vi "WhitePlot.vi"(11 "Paths":path[](array[path])=[path "/Users/crogers/Desktop/Ted/Ob16 Galahue Plowden 2013 H_Ave.trf"]) -> ()   [LabVIEW 2022 SP3]
uses:
  Perspective/subs/Perspective_Globals.vi
panel:
  in  "signal type":T1(ring)=enum."Sawtooth Wave"
  in  "# harmonics":i32=40
  in  "# freq":i32=48
  out "Graph":picture
  in  "Files":u16(ring) items=["1741 del G. HV 20 V_007.trf", "1741 del G. HV 20 V_007.trf", "1741 del G. HV 20 V_008.trf", "1741 del G. HV 20 V_008.trf", "1741 del G. HV 20 V_009.trf", "1741 del G. HV 20 V_009.trf", "1741 del G. HV 20 V_010.trf", "1741 del G. HV 20 V_010.trf", "1741 del G. HV 20 V_011.trf"]
  out "Slice":dbl[](graph)=[29.445158043811198, 36.55833093424573, 40.44091855599027, 37.67653983236719, 3.901363084528417, 43.245886090198724, 36.36206724043218, 58.6607561868737, 51.19267039727471, 16.66678219935681, 46.372145605984485, 40.65058675099788, -0.1217403502671347, 38.33577783712102, 35.852538445709634, 29.35326642077404, 49.768103526439276, 44.09040502089316, 26.44794576028672, 43.78480234185166, 12.786831883362723, nan, nan, nan, nan, nan, nan, nan, nan, nan, nan, nan, nan, nan, nan, nan, nan, nan, nan, nan]
  in  "Smoothing":u16(ring) items=["No smoothing"=0, "1/4 semitone"=25, "1/2 semitone"=50, "1 semitone"=100, "2 semitones"=200, "3 semitones"=300, "4 semitones"=400, "Octave"=1200]
  in  "Color Table":T2(ring)=enum."Rainbow"
  out "TRF":cluster{dbl, "df":dbl, dbl[]}(graph)={199.951171875, "df"=0.732421875, array[13381 elements]}
  out "2D Plot":dbl[][](graph)=[[nan, 20.049987226429913, 25.054902961250857, 29.445158043811198, 34.46385501795731, 44.780627225419565, 51.406191185965646, 49.67631609372249, 40.709611963732584, 38.92269108407762, 40.35029451326228, 33.055745098571954, 41.52467260523725, 39.21617102292643, 15.173302135246772, 40.695109109084115, 42.444899082336, 56.77593405896198, 51.382201329207334, 43.21477455890306, 50.80370011373546, 35.98612449368547, 47.77204513443894, 30.857881410259274, 46.643671439889445, 47.49403661581599, -1.4346363375750995, 19.0211768965106, 45.28695989710588, 40.69907700152897, 46.376353342172045, 39.045432783467874, 48.20425730785347, 35.99159002094946, 35.20324613314526, 51.91563451765467, 18.854037759092634, 37.28439063047342, -19.57168106597702, 25.22610299025189, 29.263013635587455, 30.82063676591259, 33.55395737125039, 18.19981181386353, 24.102157288646847, 39.34971755858826, 22.241809662116708, 68.52224965159985], [54.26627490024298, 47.12526752661166, 56.85500723817575, 36.55833093424573, 38.634265924869595, 51.93988341853376, 45.638032395871505, 66.45923338856223, 48.341086236955675, 44.73549896684294, 82.8746731094306, 36.13504669577988, 32.4985458705831, 38.46882120330299, 25.627379738354886, 38.640118352136994, 69.51016913200667, 47.08441844740895, 43.538098543664844, 37.74770538349388, 2.607749244145145, 35.43065545900197, 48.78584596653637, 44.50117153673708, 47.18149466094815, 37.167565780443084, -11.290057999008061, 38.82305284871714, 34.622338104545236, 45.77689163136356, 27.988762535569126, 35.05040002787151, 46.39143083402964, 41.744798474139316, 32.89651926775419, 62.34466322011301, 39.44356696797309, 46.6442728756223, -10.828073640077598, 26.81232522566393, 48.71727144928745, 32.03610040569839, 72.79095309960253, 36.67913423432094, 48.058266713190754, nan, nan, nan], [53.04185758812355, 84.71388448770111, 17.51080377410179, 40.44091855599027, 39.91331658353087, 28.362665427675545, 55.229556863313356, 56.42371074485528, 47.76931799964777, 39.97049168305633, 57.15726261780386, 37.542352295940155, 44.21162796738528, 17.48325982608004, 40.43782874904303, 38.742739205630784, 46.032627402046785, 20.05630274646011, 45.78665416858822, 35.24520049827762, 39.158716639789034, 11.924005690223789, 29.897529283546916, 33.60264045829483, 31.392790303731708, 19.506700819440113, -9.215795080095525, 50.42813350565264, 32.59479614372741, 31.01757424069985, 42.71237559822864, 51.983617982184924, 34.35731157695301, 42.627623260331376, 19.10147623463881, 54.50616438544329, 18.296402637224976, 58.61753732987064, nan, nan, nan, nan, nan, nan, nan, nan, nan, nan], [39.51596652723599, 29.184271442763787, 16.957827346664814, 37.67653983236719, 63.59782300125275, 48.322834414258296, 40.39060448678149, 38.07851466585304, 52.219678596166396, 61.51482106592874, 46.8634576004301, 37.06553982367735, 38.09179565041872, 11.208063972191031, 54.731123202538576, 29.039234290370757, 34.051601948841004, 41.1260225901982, 52.08899147984912, 28.05180790327435, 34.07973803463468, 42.3996411700281, 20.192703080247497, 56.168607595418976, 33.25620455392025, 39.61259618090587, 1.6416847986202243, 24.841476380656804, 37.55245428572219, 27.459839855335257, 66.77063240632266, 36.5729389128255, 41.814287416945945, nan, nan, nan, nan, nan, nan, nan, nan, nan, nan, nan, nan, nan, nan, nan], [48.16850062624863, 42.24542108686359, 44.340073178907026, 3.901363084528417, 42.347676492963295, 41.98102702804944, 32.095730941153256, 7.619084984059836, 32.35066397625168, 32.29142786493228, 40.21124807070387, 14.63732432854075, 64.87319042636963, 3.8937001997797758, 42.35230450100133, 14.130476829463692, 28.642057668910525, 38.68345012614008, 40.520552066845205, 52.826865227382584, 27.4036034714791, 73.37393650330726, 10.947826509906172, 39.440434175724384, 31.785624530969287, 39.726239419396016, 27.00365963632292, 17.381561857680012, 36.93147689751727, nan, nan, nan, nan, nan, nan, nan, nan, nan, nan, nan, nan, nan, nan, nan, nan, nan, nan, nan], [35.60423156346238, 46.08009523979531, 36.87411957248013, 43.245886090198724, 41.3473179130062, 26.344792341973875, 41.08933756077456, 27.303763144444684, 32.28100773510765, 34.38861713258833, 31.00322874795537, 55.966772111396814, 33.80384369988236, 22.921989435884473, 8.945740357752978, 42.39269732229077, 33.87217699897191, 33.14532562541018, 33.524294370197566, 44.041506495823185, 37.757502066680686, 41.939614181516674, 8.546073278104322, 48.000016608061514, 35.00765134648421, 51.85386377302325, nan, nan, nan, nan, nan, nan, nan, nan, nan, nan, nan, nan, nan, nan, nan, nan, nan, nan, nan, nan, nan, nan], [32.61310636745673, 38.97527846530624, 35.641622198785086, 36.36206724043218, 27.795949148894337, 54.187637574190326, 36.401734072540044, 30.917571343879366, 37.20179247250486, 27.793291744454113, 25.775060428523826, 10.666225801452157, 38.49962709844564, 11.781027471364073, 13.761017548356374, 42.53126220573978, 35.128829087408405, 40.161072813389424, 41.09343386515138, 35.9780075897034, 17.001024691654287, 42.92404272966259, 26.64675831650957, nan, nan, nan, nan, nan, nan, nan, nan, nan, nan, nan, nan, nan, nan, nan, nan, nan, nan, nan, nan, nan, nan, nan, nan, nan], [29.681571025848356, 42.60929144128346, 48.67052729500847, 58.6607561868737, 33.95354038216709, 41.11614535668331, 47.65431912163869, -11.009770350280277, 36.94947500875874, 39.83841719056124, 31.381560080516877, 52.500057048302736, 38.174458325750436, 20.80842003831775, 12.283677007960899, 35.16227099829001, 59.770944975043896, 21.937359659167246, 60.53209358540707, 36.682904986845664, 39.7581113435772, nan, nan, nan, nan, nan, nan, nan, nan, nan, nan, nan, nan, nan, nan, nan, nan, nan, nan, nan, nan, nan, nan, nan, nan, nan, nan, nan], [40.464054607466934, 37.58597485171173, 39.87038706581357, 51.19267039727471, 37.67639985297179, 23.13937723997912, 37.55595835553924, 42.4209222579333, 42.27910760517511, 30.522265980669758, 26.136408931304445, -2.9872106006803496, 31.322538117444275, 2.9044348449634656, 3.5797530867064515, 50.092277015634636, 38.50977087060315, 47.533818499292835, 35.62939006713031, nan, nan, nan, nan, nan, nan, nan, nan, nan, nan, nan, nan, nan, nan, nan, nan, nan, nan, nan, nan, nan, nan, nan, nan, nan, nan, nan, nan, nan], [58.5659239452997, 26.982848813621306, 36.31906856692317, 16.66678219935681, 49.49109923197512, 40.11411668922503, 37.75341628139453, 48.30992190831356, 49.081010121114915, 61.181425385472934, 22.430170217674966, 48.6155340973561, 32.675460627661636, 13.916675441379617, 21.021585447450946, 49.25166283256742, 62.27105544588605, nan, nan, nan, nan, nan, nan, nan, nan, nan, nan, nan, nan, nan, nan, nan, nan, nan, nan, nan, nan, nan, nan, nan, nan, nan, nan, nan, nan, nan, nan, nan], [54.412382522142494, 36.137207842053776, 2.764148858981666, 46.372145605984485, 37.243085887419376, 34.537737023825855, 55.257207308976035, 51.464533050016435, 39.80085824725523, 44.11810710124637, 34.10663843132296, 5.979096794947166, 25.782557120064702, 30.561510305365577, 40.94721364933057, nan, nan, nan, nan, nan, nan, nan, nan, nan, nan, nan, nan, nan, nan, nan, nan, nan, nan, nan, nan, nan, nan, nan, nan, nan, nan, nan, nan, nan, nan, nan, nan, nan], [31.369910198236113, 37.07152928092298, 10.648427094010238, 40.65058675099788, 23.51231403437172, 27.206691169768323, 36.277462506216686, 34.08022467450811, 35.763375497264654, 29.232268970303785, 23.380681094116376, 44.186129447967446, 35.05238954844841, 50.27126063942963, nan, nan, nan, nan, nan, nan, nan, nan, nan, nan, nan, nan, nan, nan, nan, nan, nan, nan, nan, nan, nan, nan, nan, nan, nan, nan, nan, nan, nan, nan, nan, nan, nan, nan], [47.82026138668182, 33.43812207351204, 25.299758140785883, -0.1217403502671347, 22.16453525325594, 48.48725544404082, 42.08447575914906, 19.62567783478579, 38.80170108501365, 40.192102073325636, 33.03273363219364, 36.03429599678489, 28.409628306750335, nan, nan, nan, nan, nan, nan, nan, nan, nan, nan, nan, nan, nan, nan, nan, nan, nan, nan, nan, nan, nan, nan, nan, nan, nan, nan, nan, nan, nan, nan, nan, nan, nan, nan, nan], [38.74276193034642, 51.348432885653914, 32.25091267120466, 38.33577783712102, 29.752691953524675, 38.079351040376174, 38.87949376223, 0.26530157389657355, 29.509618670886084, 40.33082643082275, 34.24093489901787, nan, nan, nan, nan, nan, nan, nan, nan, nan, nan, nan, nan, nan, nan, nan, nan, nan, nan, nan, nan, nan, nan, nan, nan, nan, nan, nan, nan, nan, nan, nan, nan, nan, nan, nan, nan, nan], [38.005167377161804, 31.69088276912158, 52.845640027356204, 35.852538445709634, 43.1225994596063, 37.243651148967345, 29.029508255433182, 9.006139857266586, 38.32944523498376, 36.834360308878054, nan, nan, nan, nan, nan, nan, nan, nan, nan, nan, nan, nan, nan, nan, nan, nan, nan, nan, nan, nan, nan, nan, nan, nan, nan, nan, nan, nan, nan, nan, nan, nan, nan, nan, nan, nan, nan, nan], [35.90269660816785, 39.364578709379494, 39.55419749173399, 29.35326642077404, 53.69867614237862, 31.967502560639367, 54.7193336975603, 30.88778141801589, 39.34981484445568, nan, nan, nan, nan, nan, nan, nan, nan, nan, nan, nan, nan, nan, nan, nan, nan, nan, nan, nan, nan, nan, nan, nan, nan, nan, nan, nan, nan, nan, nan, nan, nan, nan, nan, nan, nan, nan, nan, nan], [36.30638411087302, 25.09057920682725, 45.46164717529554, 49.768103526439276, 23.289405968677816, 49.15198590837125, 35.1560324577208, 42.864683043159424, nan, nan, nan, nan, nan, nan, nan, nan, nan, nan, nan, nan, nan, nan, nan, nan, nan, nan, nan, nan, nan, nan, nan, nan, nan, nan, nan, nan, nan, nan, nan, nan, nan, nan, nan, nan, nan, nan, nan, nan], [31.462436582201292, 30.362788351721534, 36.81834627839507, 44.09040502089316, 33.57068005060175, 32.74557557265104, 39.515790233414656, nan, nan, nan, nan, nan, nan, nan, nan, nan, nan, nan, nan, nan, nan, nan, nan, nan, nan, nan, nan, nan, nan, nan, nan, nan, nan, nan, nan, nan, nan, nan, nan, nan, nan, nan, nan, nan, nan, nan, nan, nan], [34.58411077100862, 33.23559013285732, -5.662822029697699, 26.44794576028672, 35.487431815874324, 40.942138140629154, nan, nan, nan, nan, nan, nan, nan, nan, nan, nan, nan, nan, nan, nan, nan, nan, nan, nan, nan, nan, nan, nan, nan, nan, nan, nan, nan, nan, nan, nan, nan, nan, nan, nan, nan, nan, nan, nan, nan, nan, nan, nan], [34.61465926871371, 17.18392844569568, 13.031570274998831, 43.78480234185166, 56.1573881112846, nan, nan, nan, nan, nan, nan, nan, nan, nan, nan, nan, nan, nan, nan, nan, nan, nan, nan, nan, nan, nan, nan, nan, nan, nan, nan, nan, nan, nan, nan, nan, nan, nan, nan, nan, nan, nan, nan, nan, nan, nan, nan, nan], [29.186029345513607, 47.978737915500574, 17.360000383750858, 12.786831883362723, nan, nan, nan, nan, nan, nan, nan, nan, nan, nan, nan, nan, nan, nan, nan, nan, nan, nan, nan, nan, nan, nan, nan, nan, nan, nan, nan, nan, nan, nan, nan, nan, nan, nan, nan, nan, nan, nan, nan, nan, nan, nan, nan, nan], [25.72159338389789, 36.84666611970028, 34.76691669928632, nan, nan, nan, nan, nan, nan, nan, nan, nan, nan, nan, nan, nan, nan, nan, nan, nan, nan, nan, nan, nan, nan, nan, nan, nan, nan, nan, nan, nan, nan, nan, nan, nan, nan, nan, nan, nan, nan, nan, nan, nan, nan, nan, nan, nan], [27.424976418713154, 38.48369817799687, 50.658137928834435, nan, nan, nan, nan, nan, nan, nan, nan, nan, nan, nan, nan, nan, nan, nan, nan, nan, nan, nan, nan, nan, nan, nan, nan, nan, nan, nan, nan, nan, nan, nan, nan, nan, nan, nan, nan, nan, nan, nan, nan, nan, nan, nan, nan, nan], [34.75082504002703, 44.286747839093266, nan, nan, nan, nan, nan, nan, nan, nan, nan, nan, nan, nan, nan, nan, nan, nan, nan, nan, nan, nan, nan, nan, nan, nan, nan, nan, nan, nan, nan, nan, nan, nan, nan, nan, nan, nan, nan, nan, nan, nan, nan, nan, nan, nan, nan, nan], [35.40073024186071, nan, nan, nan, nan, nan, nan, nan, nan, nan, nan, nan, nan, nan, nan, nan, nan, nan, nan, nan, nan, nan, nan, nan, nan, nan, nan, nan, nan, nan, nan, nan, nan, nan, nan, nan, nan, nan, nan, nan, nan, nan, nan, nan, nan, nan, nan, nan], [28.955349958389448, nan, nan, nan, nan, nan, nan, nan, nan, nan, nan, nan, nan, nan, nan, nan, nan, nan, nan, nan, nan, nan, nan, nan, nan, nan, nan, nan, nan, nan, nan, nan, nan, nan, nan, nan, nan, nan, nan, nan, nan, nan, nan, nan, nan, nan, nan, nan], [nan, nan, nan, nan, nan, nan, nan, nan, nan, nan, nan, nan, nan, nan, nan, nan, nan, nan, nan, nan, nan, nan, nan, nan, nan, nan, nan, nan, nan, nan, nan, nan, nan, nan, nan, nan, nan, nan, nan, nan, nan, nan, nan, nan, nan, nan, nan, nan], [nan, nan, nan, nan, nan, nan, nan, nan, nan, nan, nan, nan, nan, nan, nan, nan, nan, nan, nan, nan, nan, nan, nan, nan, nan, nan, nan, nan, nan, nan, nan, nan, nan, nan, nan, nan, nan, nan, nan, nan, nan, nan, nan, nan, nan, nan, nan, nan], [nan, nan, nan, nan, nan, nan, nan, nan, nan, nan, nan, nan, nan, nan, nan, nan, nan, nan, nan, nan, nan, nan, nan, nan, nan, nan, nan, nan, nan, nan, nan, nan, nan, nan, nan, nan, nan, nan, nan, nan, nan, nan, nan, nan, nan, nan, nan, nan], [nan, nan, nan, nan, nan, nan, nan, nan, nan, nan, nan, nan, nan, nan, nan, nan, nan, nan, nan, nan, nan, nan, nan, nan, nan, nan, nan, nan, nan, nan, nan, nan, nan, nan, nan, nan, nan, nan, nan, nan, nan, nan, nan, nan, nan, nan, nan, nan], [nan, nan, nan, nan, nan, nan, nan, nan, nan, nan, nan, nan, nan, nan, nan, nan, nan, nan, nan, nan, nan, nan, nan, nan, nan, nan, nan, nan, nan, nan, nan, nan, nan, nan, nan, nan, nan, nan, nan, nan, nan, nan, nan, nan, nan, nan, nan, nan], [nan, nan, nan, nan, nan, nan, nan, nan, nan, nan, nan, nan, nan, nan, nan, nan, nan, nan, nan, nan, nan, nan, nan, nan, nan, nan, nan, nan, nan, nan, nan, nan, nan, nan, nan, nan, nan, nan, nan, nan, nan, nan, nan, nan, nan, nan, nan, nan], [nan, nan, nan, nan, nan, nan, nan, nan, nan, nan, nan, nan, nan, nan, nan, nan, nan, nan, nan, nan, nan, nan, nan, nan, nan, nan, nan, nan, nan, nan, nan, nan, nan, nan, nan, nan, nan, nan, nan, nan, nan, nan, nan, nan, nan, nan, nan, nan], [nan, nan, nan, nan, nan, nan, nan, nan, nan, nan, nan, nan, nan, nan, nan, nan, nan, nan, nan, nan, nan, nan, nan, nan, nan, nan, nan, nan, nan, nan, nan, nan, nan, nan, nan, nan, nan, nan, nan, nan, nan, nan, nan, nan, nan, nan, nan, nan], [nan, nan, nan, nan, nan, nan, nan, nan, nan, nan, nan, nan, nan, nan, nan, nan, nan, nan, nan, nan, nan, nan, nan, nan, nan, nan, nan, nan, nan, nan, nan, nan, nan, nan, nan, nan, nan, nan, nan, nan, nan, nan, nan, nan, nan, nan, nan, nan], [nan, nan, nan, nan, nan, nan, nan, nan, nan, nan, nan, nan, nan, nan, nan, nan, nan, nan, nan, nan, nan, nan, nan, nan, nan, nan, nan, nan, nan, nan, nan, nan, nan, nan, nan, nan, nan, nan, nan, nan, nan, nan, nan, nan, nan, nan, nan, nan], [nan, nan, nan, nan, nan, nan, nan, nan, nan, nan, nan, nan, nan, nan, nan, nan, nan, nan, nan, nan, nan, nan, nan, nan, nan, nan, nan, nan, nan, nan, nan, nan, nan, nan, nan, nan, nan, nan, nan, nan, nan, nan, nan, nan, nan, nan, nan, nan], [nan, nan, nan, nan, nan, nan, nan, nan, nan, nan, nan, nan, nan, nan, nan, nan, nan, nan, nan, nan, nan, nan, nan, nan, nan, nan, nan, nan, nan, nan, nan, nan, nan, nan, nan, nan, nan, nan, nan, nan, nan, nan, nan, nan, nan, nan, nan, nan], [nan, nan, nan, nan, nan, nan, nan, nan, nan, nan, nan, nan, nan, nan, nan, nan, nan, nan, nan, nan, nan, nan, nan, nan, nan, nan, nan, nan, nan, nan, nan, nan, nan, nan, nan, nan, nan, nan, nan, nan, nan, nan, nan, nan, nan, nan, nan, nan], [nan, nan, nan, nan, nan, nan, nan, nan, nan, nan, nan, nan, nan, nan, nan, nan, nan, nan, nan, nan, nan, nan, nan, nan, nan, nan, nan, nan, nan, nan, nan, nan, nan, nan, nan, nan, nan, nan, nan, nan, nan, nan, nan, nan, nan, nan, nan, nan]]
  out "size(s)":i32=65
  # "Plotting Energy At Overtones"
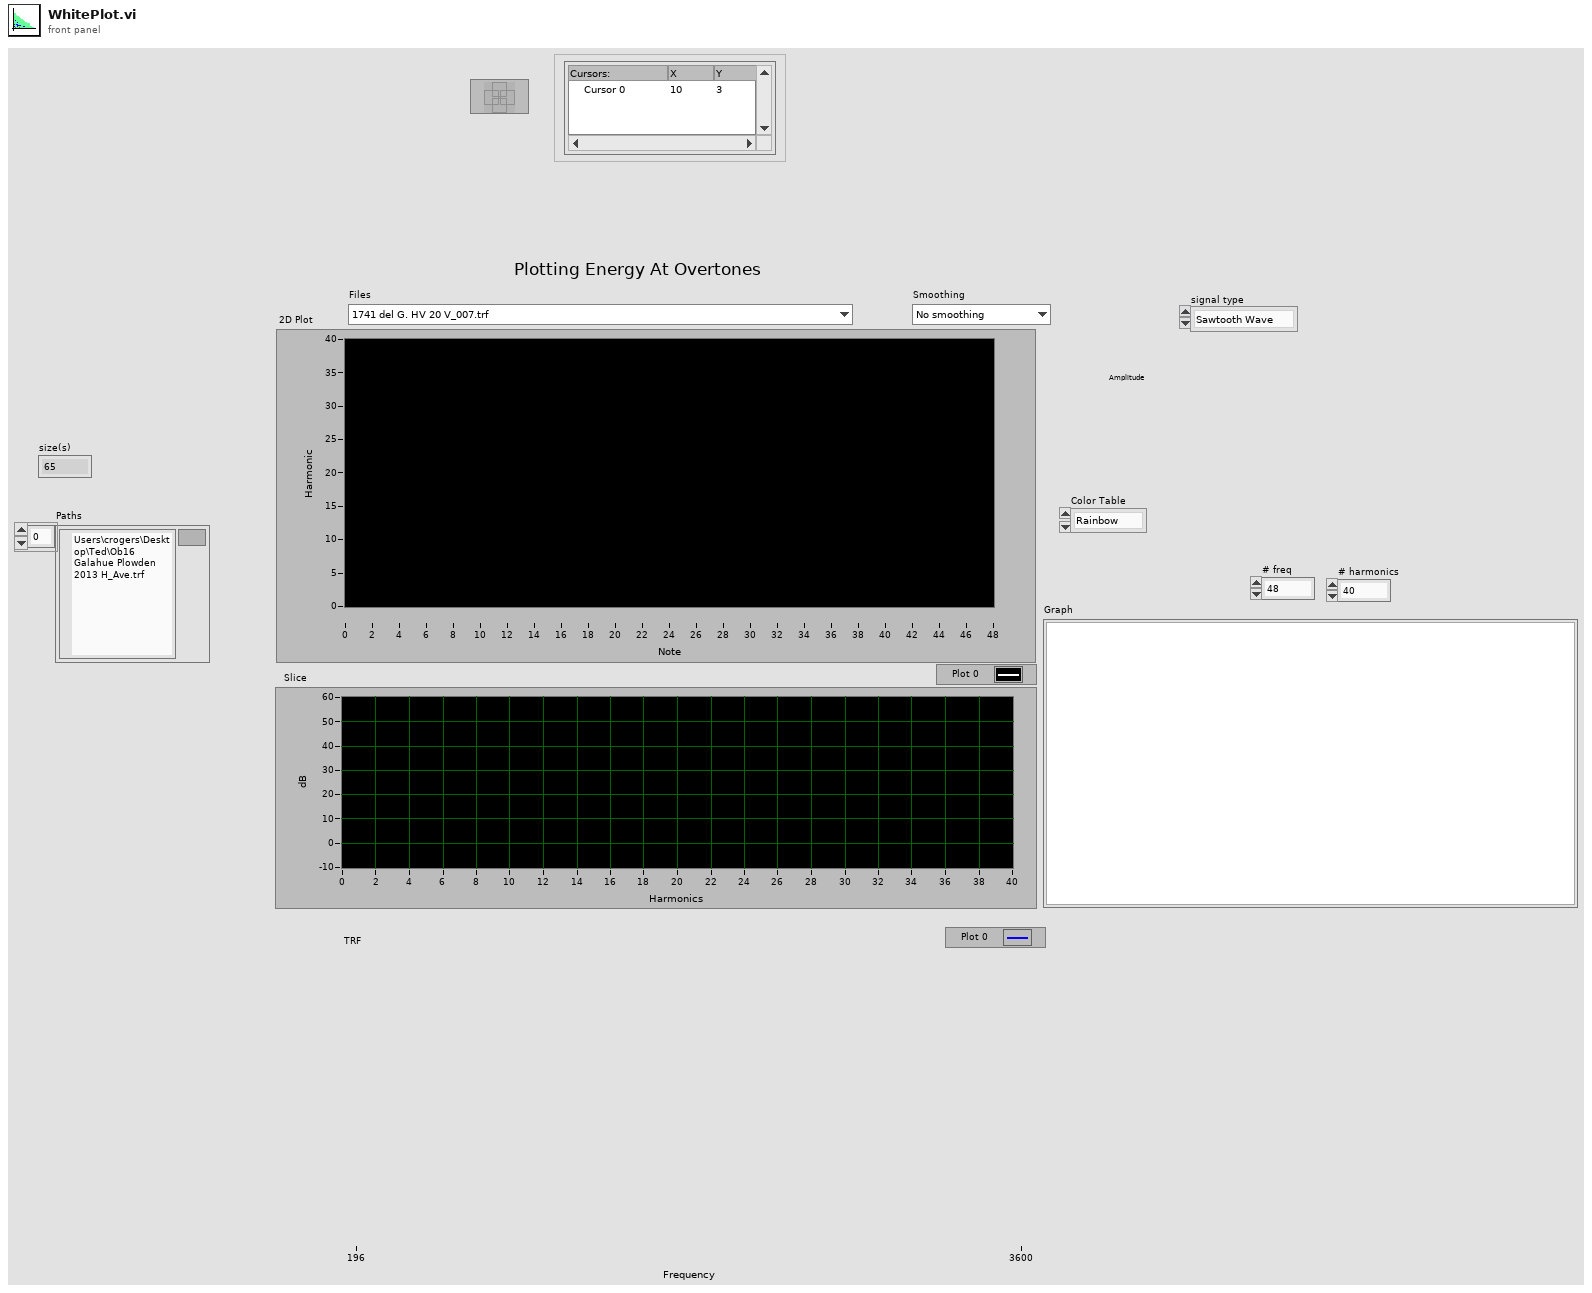
[diagram p1: front panel]
types:
  T1 = enum16{"Sine Wave", "Triangle Wave", "Square Wave", "Sawtooth Wave"}
  T2 = enum16{"Apricot", "Carnation", "Ether", "Greyscale", "Greyscale-banded", "Hot Metal", "Lava Waves", "Mac", "Morning Glory", "Rainbow", "Rainbow-banded", "Rainbow-inverted", "Rainbow-striped", "Saturn", "Seismic", "Space"}
  T3 = cluster{"Notes":string, "format string":string}[]
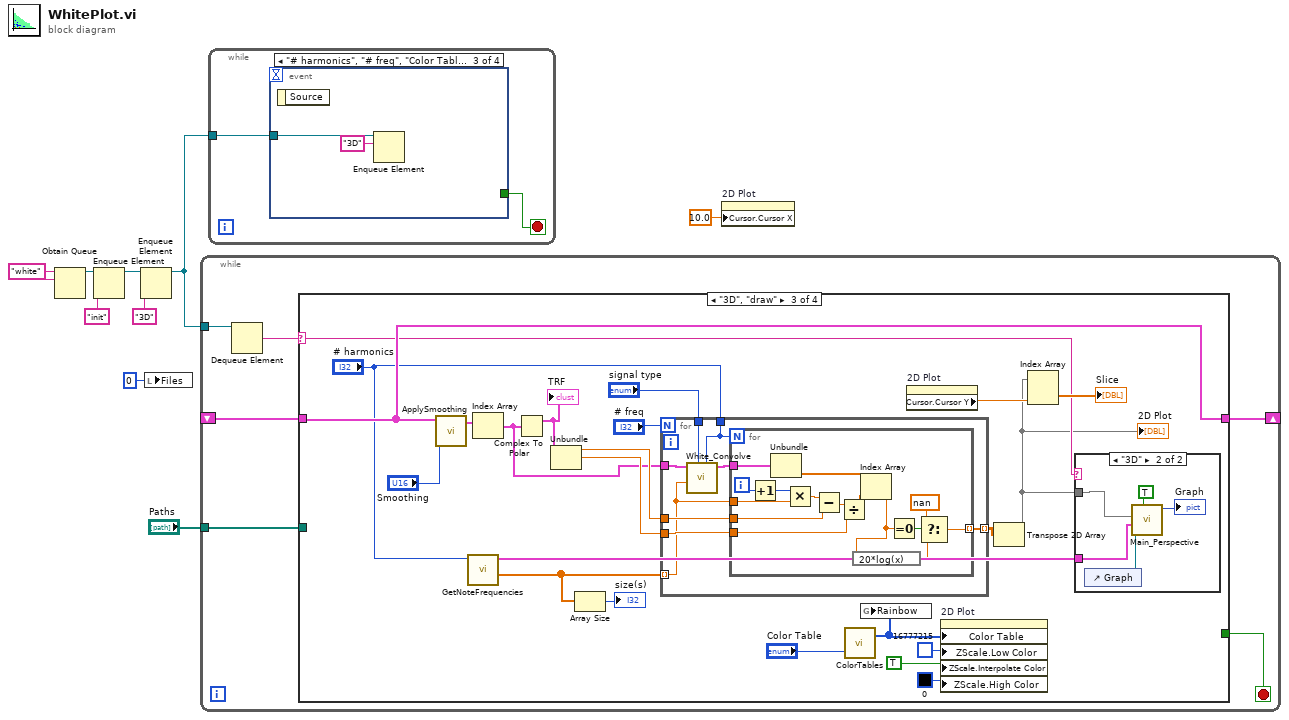
[diagram p0: block diagram]
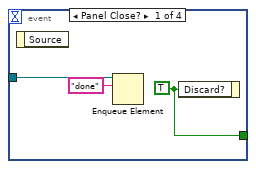
[diagram p2: hidden frame]
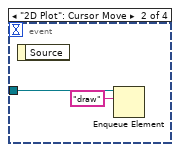
[diagram p3: hidden frame]
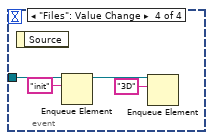
[diagram p4: hidden frame]
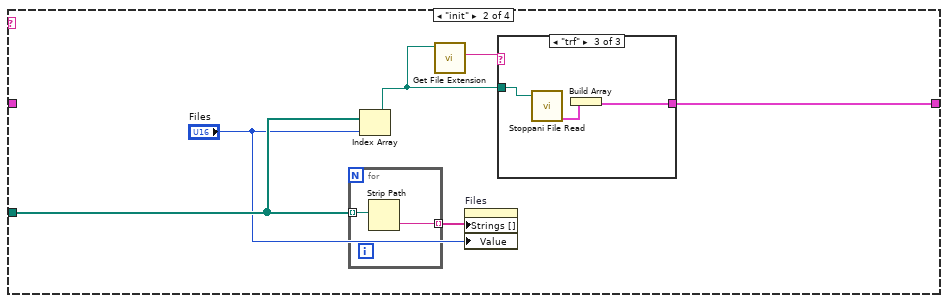
[diagram p6: hidden frame]
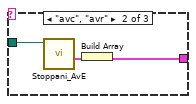
[diagram p8: hidden frame]
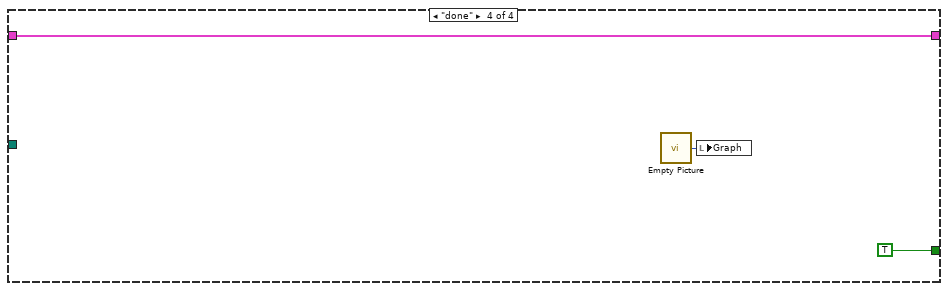
[diagram p10: hidden frame]
diagram:
  w9 = "white" ("name (unnamed)")
  n1 = Obtain Queue(name (unnamed)=w9, element data type=w9) -> (queue out=w5:refnum<queue>)  [unwired: 3 in, 2 out]
  n2 = Enqueue Element(queue=w5, element="init") -> (queue out=w4:refnum<queue>)  [unwired: 2 in, 2 out]
  n3 = Enqueue Element(queue=w4, element="3D") -> (queue out=w8:refnum<queue>)  [unwired: 2 in, 2 out]
  n4 = local write "Files"(0) -> ()
  n5 = while {
    tunnel: w8 -> [w15]
    shift-right: [w11] -> _
    shift-left: _ -> [w12]
    tunnel: "Paths" -> [w10]
    stop <- w13 stop-if-true
    n6 = Dequeue Element(queue=w15) -> (element=w14:string)  [unwired: 2 in, 3 out]
    n7 = case shown="\"3D\", \"draw\"" w14 {
      selector: w14 -> [_ _ w40 _]
      tunnel: [_ _ _ TRUE ("Discard?")] -> w13
      tunnel: w12 -> [w16 _ w43 w83]
      tunnel: [w16 w21 w43 w83] -> w11
      tunnel: w10 -> [_ w20 _ _]
      frame Default {
      }
      frame "init" {
        n8 = for {
          tunnel: w20 -> [w30] mode=indexing
          tunnel: [w29] -> w22 mode=indexing
          n9 = Strip Path(path=w30) -> (name=w29:string)  [unwired: 1 out]
        }
        n10 = Index Array(array=w20, index="Files") -> (element=w18:path)
        n11 = call <vilib>:"Get File Extension.vi"("file"=w18) -> ("lowercase file extension"=w17:string)  [unwired: 6 in, 4 out]
        n12 = property on="Files" class="Ring (strict)"("Strings []"=w22, "Value"="Files") -> ()  [unwired: 2 in, 2 out]
        n13 = case shown="\"trf\"" w17 {
          tunnel: w18 -> [_ w25 w27]
          tunnel: [_ w23 w28] -> w21
          frame Default {
          }
          frame "avc", "avr" {
            n14 = call "Stoppani_AvE.vi"("file (use dialog)"=w25) -> ("Complex FRF"=w24:cluster{"t0":dbl, "df":dbl, "Y":cdb[]})  [unwired: 7 in, 3 out]
            n15 = Build Array(w24) -> (w23:cluster{"t0":dbl, "df":dbl, "Y":cdb[]}[])
          }
          frame "trf" {
            n16 = call "Stoppani File Read.vi"("String in"=w27) -> ("Complex FRF"=w26:cluster{"t0":dbl, "dt":dbl, "Y":cdb[]})  [unwired: 2 in, 3 out]
            n17 = Build Array(w26) -> (w28:cluster{"t0":dbl, "dt":dbl, "Y":cdb[]}[])
          }
        }
      }
      frame "3D", "draw" {
        n18 = call "ApplySmoothing.vi"("Smoothing"="Smoothing", "Complex FRF"=w43) -> ("Complex FRF Out"=w50:cluster{dbl, "df":dbl, cdb[]}[])  [unwired: 9 in]
        n19 = call "GetNoteFrequencies.vi"("# harmonics"="# harmonics") -> ("frequencies"=w32:dbl[], "Labels"=w31:T3)  [unwired: 8 in, 1 out]
        n20 = Index Array(array=w50) -> (element=w34:cluster{dbl, "df":dbl, cdb[]})  [unwired: 1 in]
        n21 = Complex To Polar(r * e^(i*theta)=w34) -> (r=w51:cluster{dbl, "df":dbl, dbl[]})  [unwired: 1 out]
        "TRF" <- w51
        n22 = Unbundle(w51) -> (w52:dbl, "df"=w36:dbl)  [unwired: 1 out]
        n23 = Array Size(array=w32) -> (size(s)=→"size(s)":i32)
        n24 = for {
          N: "# freq" -> [_]
          tunnel: w34 -> [w62]
          tunnel: [w64] -> w39 mode=indexing
          tunnel: w32 -> [w61] mode=indexing
          tunnel: w52 -> [w65]
          tunnel: w36 -> [w66]
          tunnel: "# harmonics" -> [w59]
          tunnel: "signal type" -> [w60]
          n25 = call "White_Convolve.vi"("# harmonics"=w59, "signal type"=w60, "frequency"=w61, "Complex FRF"=w62) -> ("convolution"=w63:cluster{dbl, "df":dbl, dbl[]})  [unwired: 7 in]
          n26 = for {
            N: w59 -> [_]
            tunnel: w63 -> [w81]
            tunnel: w61 -> [w77]
            tunnel: w65 -> [w76]
            tunnel: w66 -> [w75]
            tunnel: [w71] -> w64 mode=indexing
            i -> [w73]
            n27 = Increment(x=w73) -> (x+1=w80:i32)
            n28 = Unbundle(w81) -> (w67:dbl[])  [unwired: 2 out]
            n29 = Multiply(x=w80, y=w77) -> (x*y=w79:dbl)
            n30 = Subtract(x=w79, y=w76) -> (x-y=w78:dbl)
            n31 = Divide(x=w78, y=w75) -> (x/y=w74:dbl)
            n32 = Index Array(array=w67, index=w74) -> (element=w69:dbl)
            n33 = expression code="20*log(x)"(w69) -> (w68:dbl)
            n34 = Equal To 0?(x=w69) -> (x = 0?=w72:bool)
            n35 = Select(t=nan, s=w72, f=w68) -> (s? t:f=w71:dbl)
          }
        }
        n36 = call "ColorTables.vi"("Color Table"="Color Table") -> ("Color Table Out"=w41:u32[])  [unwired: 2 in]
        n37 = global write "Perspective_Globals.vi" "Rainbow"(w41) -> ()
        n38 = property on="2D Plot" class="IntGraph (strict)"() -> ("Cursor.Cursor Y"=w38:dbl)  [unwired: 2 in, 2 out]
        n39 = property on="2D Plot" class="IntGraph (strict)"("Color Table"=w41, "ZScale.Low Color"=u32 16777215 ("Z Scale.Low Color"), "ZScale.Interpolate Color"=TRUE ("Z Scale.Interpolate Color"), "ZScale.High Color"=u32 0 ("Z Scale.High Color")) -> ()  [unwired: 2 in, 2 out]
        n40 = Transpose 2D Array(2D array=w39) -> (transposed array=w37:dbl[][])
        "2D Plot" <- w37
        n41 = Index Array(array=w37, index (col)=w38) -> (element=→"Slice":dbl[])  [unwired: 1 in]
        n42 = case shown="\"3D\"" w40 {
          tunnel: w37 -> [_ w55]
          tunnel: w31 -> [_ w56]
          frame "False", Default {
          }
          frame "3D" {
            n43 = control-ref of="Graph"() -> (w54:refnum<vi>)
            n44 = call "Main_Perspective.vi"("3D?"=TRUE, "reference"=w54, "labels"=w56, "White Plot"=w55) -> ("Graph"=→"Graph":picture)  [unwired: 7 in]
          }
        }
      }
      frame "done" {
        n45 = call "Empty Picture"() -> ("empty picture"=w82:picture)
        n46 = local write "Graph"(w82) -> ()
      }
    }
  }
  n47 = while {
    tunnel: w8 -> [w86]
    stop <- w85 stop-if-true
    n48 = event shown="[2] \"# harmonics\", \"# freq\", \"Color Table\", \"Smoothing\", \"signal type\": Value Change" {
      selector: _ -> [_ _ _ _]
      dyn-events: _ -> [_ _ _ _]
      timeout: _ -> [_ _ _ _]
      tunnel: w86 -> [w89 w91 w93 w97]
      tunnel: [w87 _ _ _] -> w85
      event Panel Close? {
        w87 = TRUE ("Discard?")
        n49 = event-data() -> ()  [unwired: 1 in, 1 out]
        n50 = Enqueue Element(queue=w89, element="done") -> ()  [unwired: 2 in, 3 out]
        n51 = event-data("Discard?"=w87) -> ()  [unwired: 1 in, 1 out]
      }
      event "2D Plot": Cursor Move {
        n52 = event-data() -> ()  [unwired: 1 in, 1 out]
        n53 = Enqueue Element(queue=w91, element="draw") -> ()  [unwired: 2 in, 3 out]
      }
      event "# harmonics", "# freq", "Color Table", "Smoothing", "signal type": Value Change {
        n54 = event-data() -> ()  [unwired: 1 in, 1 out]
        n55 = Enqueue Element(queue=w93, element="3D") -> ()  [unwired: 2 in, 3 out]
      }
      event "Files": Value Change {
        n56 = event-data() -> ()  [unwired: 1 in, 1 out]
        n57 = Enqueue Element(queue=w97, element="init") -> (queue out=w94:refnum<queue>)  [unwired: 2 in, 2 out]
        n58 = Enqueue Element(queue=w94, element="3D") -> ()  [unwired: 2 in, 3 out]
      }
    }
  }
  n59 = property on="2D Plot" class="IntGraph (strict)"("Cursor.Cursor X"=10.0 ("Cursor.Cursor Position:Cursor X")) -> ()  [unwired: 2 in, 2 out]
